vi "svl_Peak Resampled Level (1 Ch).vi"(8 "error in (no error)":errorcluster, 9 "processing state":T1(ring), 11 "even angle signal":T2 {"even angle signal" format="%.2f"; "dr" format="%.2f"; "r0" format="%.2f"}) -> (0 "error out":errorcluster, 3 "peak level":dbl format="%.2f")   [LabVIEW 2017]
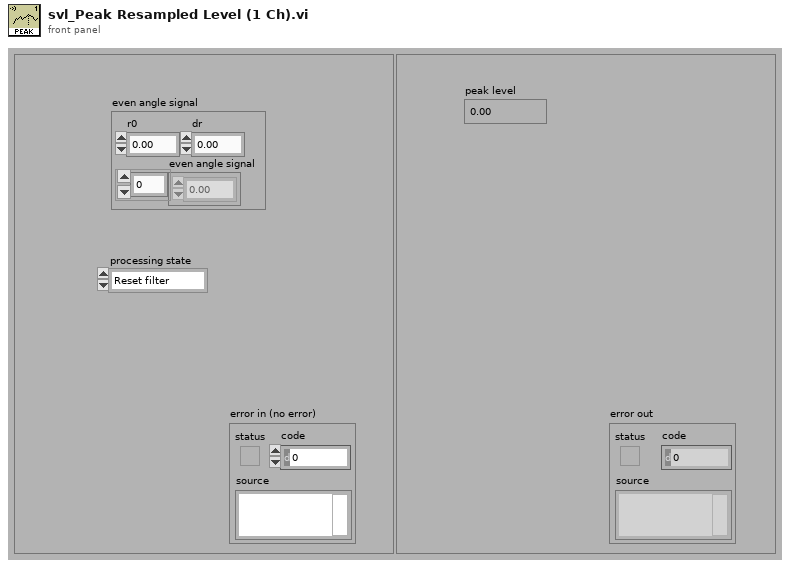
[diagram p1: front panel]
types:
  T1 = enum16{"Reset filter", "Restart averaging", "Continue processing"}
  T2 = cluster{"r0":dbl, "dr":dbl, "even angle signal":dbl[]}
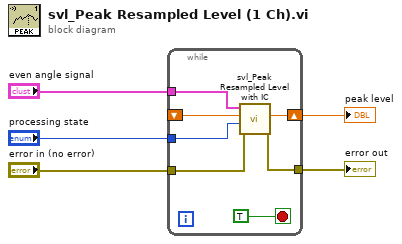
[diagram p0: block diagram]
diagram:
  n1 = while {
    shift-left: _ -> [w9]
    shift-right: [w8] -> w1
    tunnel: [w11] -> w2
    tunnel: "error in (no error)" -> [w12]
    tunnel: "processing state" -> [w7]
    tunnel: "even angle signal" -> [w6]
    stop <- TRUE stop-if-true
    n2 = call <vilib>:"svl_Peak Resampled Level with IC.vi"("error in (no error)"=w12, "processing state"=w7, "initial soundLevel"=w9, "even angle signal"=w6) -> ("error out"=w11:errorcluster, "final soundLevel"=w8:dbl)  [unwired: 6 in]
  }
  "peak level" <- w1
  "error out" <- w2
